vi "Parse Description String.vi"(8 "error in (no error)":errorcluster, 11 "Description String":string) -> (0 "error out":errorcluster, 1 "Data Directory":path, 2 "Modbus Address":u8, 3 "IP Address":string, 5 "Device Type":string)   [LabVIEW 2020, in "polar_bear_plus_drivers.lvlib" / "heater_parent.lvclass"]
doc: "Parses a description string generated from the \"Generate Description String\" VI into the IP address, modbus address, and data directory path."
uses:
  <instrlib>/RxnRover/Driver Polar Bear Plus/heater_parent/heater_parent.lvclass
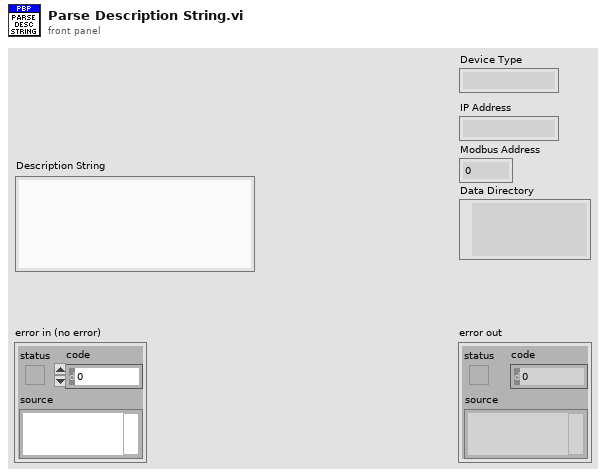
[diagram p1: front panel]
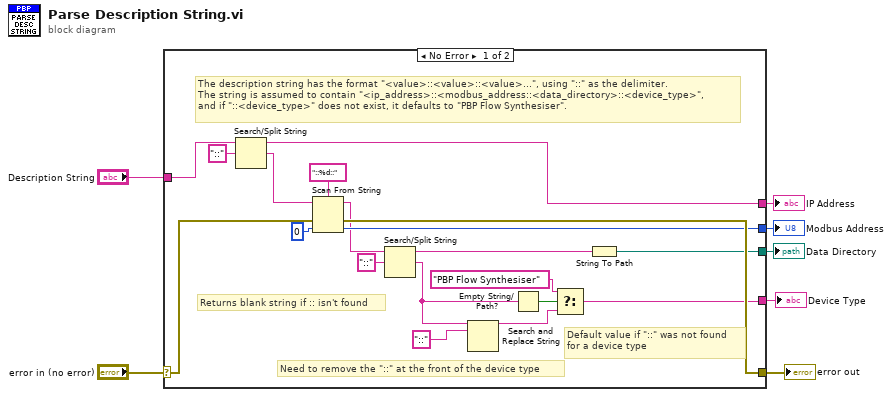
[diagram p0: block diagram]
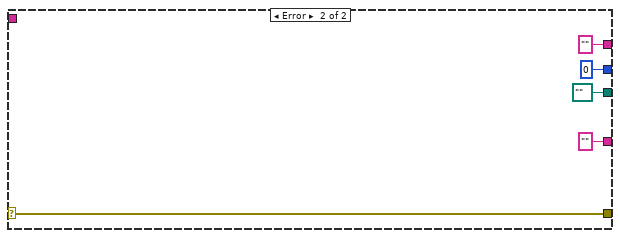
[diagram p2: hidden frame]
diagram:
  n1 = case shown="No Error" "error in (no error)" {
    selector: "error in (no error)" -> [w25 w31]
    tunnel: [w24 w31] -> w6
    tunnel: "Description String" -> [w23 _]
    tunnel: [w21 ""] -> w4
    tunnel: [w19 u8 0 ("default value 2")] -> w3
    tunnel: [w18 path ""] -> w2
    tunnel: [w11 "" ("t")] -> w1
    frame No Error {
      # "Need to remove the \"::\" at the front of the device type"
      # "Default value if \"::\" was not found\nfor a device type"
      # "The description string has the format \"<value>::<value>::<value>...\", using \"::\" as the delimiter.\nThe string is assumed to contain \"<ip_address>::<modbus_address::<data_directory>::<device_type>\",\nand if \"::<device_type>\" does not exist, it defaults to \"PBP Flow Synthesiser\"."
      # "Returns blank string if :: isn't found"
      n2 = Search/Split String(string=w23, search string/char (-)="::") -> (substring before match=w21:string, match + rest of string=w20:string)  [unwired: 1 in, 1 out]
      n3 = Scan From String(format string="::%d::", input string=w20, error in=w25, default 1=u8 0 ("default value 2")) -> (remaining string=w15:string, error out=w24:errorcluster, output 1=w19:u8)  [unwired: 1 in, 1 out]
      n4 = Search/Split String(string=w15, search string/char (-)="::") -> (substring before match=w14:string, match + rest of string=w9:string)  [unwired: 1 in, 1 out]
      n5 = Search and Replace String(input string=w9, search string="::") -> (result string=w10:string)  [unwired: 6 in, 3 out]
      n6 = Empty String/Path?(string/path=w9) -> (empty?=w13:bool)
      n7 = Select(t="PBP Flow Synthesiser", s=w13, f=w10) -> (s? t:f=w11:string)
      n8 = String To Path(string=w14) -> (path=w18:path)
    }
    frame Error {
    }
  }
  "error out" <- w6
  "IP Address" <- w4
  "Modbus Address" <- w3
  "Data Directory" <- w2
  "Device Type" <- w1
